vi "Coord window-Cross validate index of clicked FOV.vi"(11 "Coordinates of pixel clicked on":T1) -> (3 "Output Array":i32[](array[numeric]))   [LabVIEW 2013]
uses:
  <vilib>/Utility/miscctls.llb/LVPoint32TypeDef.ctl
  Globals/Coord window-Globals.vi
  Program Files (x86)/National Instruments/LabVIEW 2013/user.lib/_OpenG.lib/array/array.llb/Remove Duplicates from 1D Array (I32)__ogtk.vi
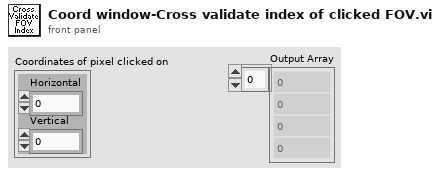
[diagram p1: front panel]
types:
  T1 = typedef "LVPoint32TypeDef.ctl" = cluster{"Horizontal":i32, "Vertical":i32}
  T2 = typedef "Coordinate list window refs.ctl" = cluster{"Window Name (i.e. Key)":string, "menu reference":refnum<k9>, "VI's reference":refnum<vi>, "Pane 1":refnum<vi>, "Pane 2":refnum<vi>, "Coord Listbox":refnum<vi>, "File name":refnum<vi>, "Picture Map":refnum<vi>, "Stage XYZ Position ind.":refnum<vi>}
  T3 = typedef "LVBoundsTypeDef.ctl" = cluster{"Width":u32, "Height":u32}
  T4 = cluster{"FOV/2-X (pixels)":i16, "FOV/2-Y (pixels)":i16}
  T5 = cluster{"left":i16, "top":i16, "right":i16, "bottom":i16}
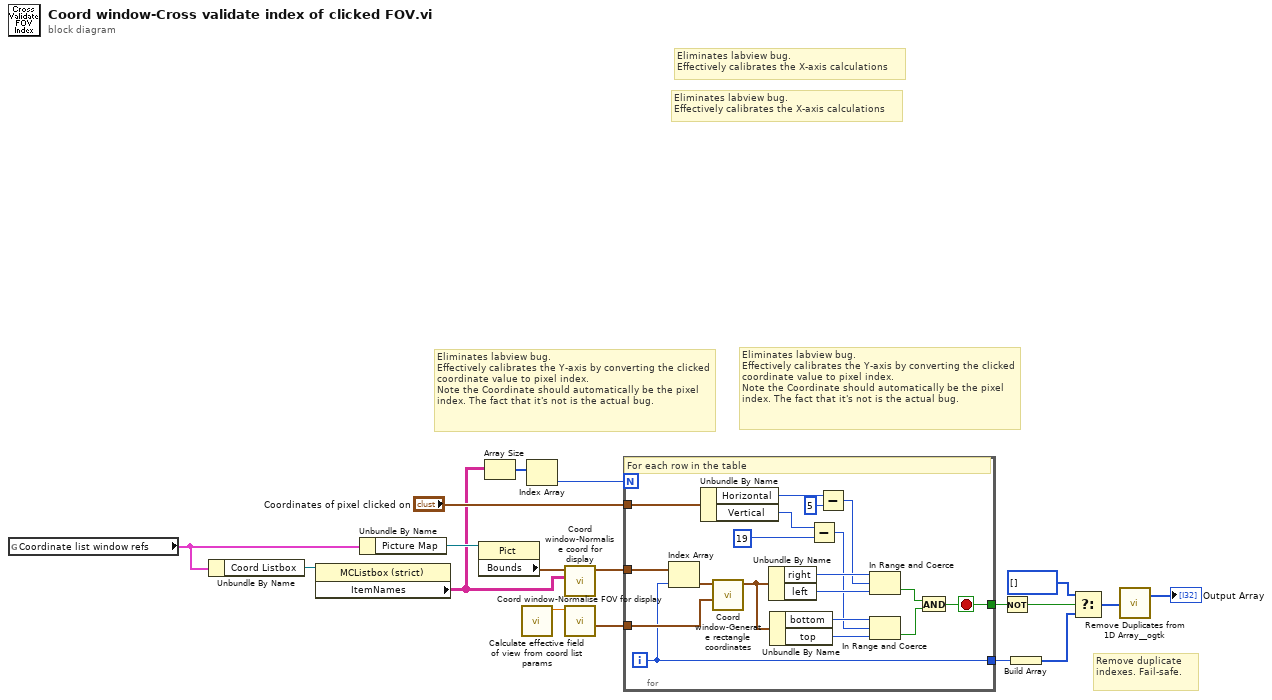
[diagram p0: block diagram]
diagram:
  # "Eliminates labview bug.\nEffectively calibrates the Y-axis by converting the clicked coordinate value to pixel index.\nNote the Coordinate should automatically be the pixel index. The fact that it's not is the actual bug."
  # "Eliminates labview bug.\nEffectively calibrates the X-axis calculations"
  # "Eliminates labview bug.\nEffectively calibrates the Y-axis by converting the clicked coordinate value to pixel index.\nNote the Coordinate should automatically be the pixel index. The fact that it's not is the actual bug."
  # "Eliminates labview bug.\nEffectively calibrates the X-axis calculations"
  # "Remove duplicate indexes. Fail-safe."
  n1 = global read "Coord window-Globals.vi" "Coordinate list window refs"() -> (w15:T2)
  n2 = Unbundle By Name(w15) -> ("Coord Listbox"=w14:refnum<vi>)
  n3 = property class="MCListbox (strict)"(reference=w14) -> ("ItemNames"=w4:string[][])  [unwired: 1 in, 2 out]
  n4 = Unbundle By Name(w15) -> ("Picture Map"=w13:refnum<vi>)
  n5 = property on="Property Node" class="Pict"(reference=w13) -> ("Bounds"=w12:T3)  [unwired: 1 in, 2 out]
  n6 = Array Size(array=w4) -> (size(s)=w3:i32[])
  n7 = call "Calculate effective field of view from coord list params.vi"() -> ("Effective FOV (um)"=w1:sgl)  [unwired: 11 in]
  n8 = Index Array(array=w3) -> (element=w2:i32)  [unwired: 1 in]
  n9 = call "Coord window-Normalise coord for display.vi"("MCList ItemNames"=w4, "Bounds"=w12) -> ("Normalised coordinates (for display)"=w10:cluster{"x":i16, "y":i16}[])  [unwired: 9 in]
  n10 = call "Coord window-Normalise FOV for display.vi"("Effective FOV (um)"=w1) -> ("Normalised Effective FOV/2"=w11:T4)  [unwired: 9 in, 1 out]
  n11 = for {
    N: w2 -> [_]
    tunnel: w10 -> [w37]
    tunnel: w11 -> [w35]
    tunnel: "Coordinates of pixel clicked on" -> [w33]
    tunnel: [w19] -> w9
    tunnel: [w20] -> w8
    i -> [w19]
    stop <- w20 stop-if-true
    # "For each row in the table"
    n12 = Index Array(array=w37, index=w19) -> (element=w36:cluster{"x":i16, "y":i16})
    n13 = Unbundle By Name(w33) -> ("Horizontal"=w23:i32, "Vertical"=w25:i32)
    n14 = call "Coord window-Generate rectangle coordinates.vi"("Normalised Effective FOV/2"=w35, "Norm point(x,y) (for display)"=w36) -> ("Norm rect (for display)"=w34:T5)  [unwired: 9 in]
    n15 = Unbundle By Name(w34) -> ("right"=w32:i16, "left"=w31:i16)
    n16 = Unbundle By Name(w34) -> ("bottom"=w30:i16, "top"=w29:i16)
    n17 = Subtract(x=w25, y=19 ("Correction offset")) -> (x-y=w24:i32)
    n18 = Subtract(x=w23, y=5) -> (x-y=w22:i32)
    n19 = In Range and Coerce(upper limit=w32, x=w22, lower limit=w31) -> (In Range?=w28:bool)  [unwired: 1 out]
    n20 = In Range and Coerce(upper limit=w30, x=w24, lower limit=w29) -> (In Range?=w27:bool)  [unwired: 1 out]
    n21 = And(x=w28, y=w27) -> (x .and. y?=w20:bool)
  }
  n22 = Not(x=w8) -> (.not. x?=w7:bool)
  n23 = Build Array(w9) -> (w5:i32[])
  n24 = Select(t=i32[] [], s=w7, f=w5) -> (s? t:f=w18:i32[])
  n25 = call-poly "Remove Duplicates from 1D Array__ogtk.vi"("Input Array"=w18) -> ("Output Array"=→"Output Array":i32[])  [unwired: 1 out]
